vi "CONFIGURE_DIGITIZER_2.vi"(0 "VERTICAL SETTINGS IN":T3, 1 "DIGITIZER 2 CHANNELS":string, 2 "Horizontal Settings IN":T1, 3 "error in":errorcluster, 4 "TRIGGER SETTINGS IN":T2) -> (5 "instrument handle out":refnum<k15>, 6 "error out":errorcluster)   [LabVIEW 2010]
uses:
  <instrlib>/niScope/Controls/niScope trigger slope.ctl
  <instrlib>/niScope/Controls/niScope trigger source.ctl
  <instrlib>/niScope/Controls/niScope trigger source digital.ctl
  <instrlib>/niScope/Configure/Trigger/niScope Configure Trigger Edge.vi
  <instrlib>/niScope/Configure/Trigger/niScope Configure Trigger Digital.vi
  <instrlib>/niScope/Configure/Trigger/niScope Configure Trigger Immediate.vi
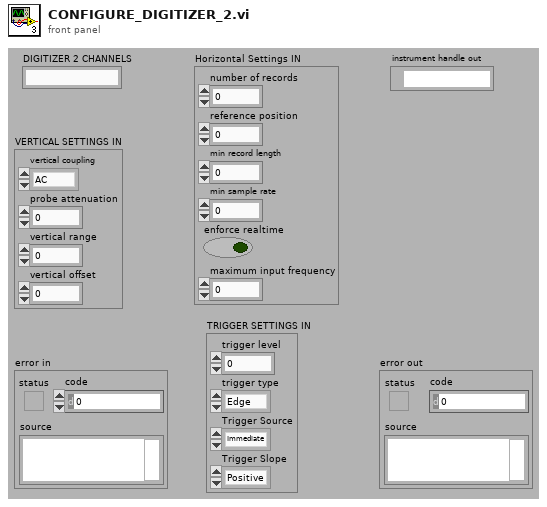
[diagram p1: front panel]
types:
  T1 = cluster{"number of records":i32, "reference position":dbl, "min record length":i32, "min sample rate":dbl, "enforce realtime":bool, "maximum input frequency":dbl}
  T2 = cluster{"trigger level":dbl, "trigger type":enum16{"Edge", "Digital", "Immediate"}, "Trigger Source":enum8{"Immediate", "Channel 0", "Channel 1", "Channel 2", "Channel 3", "Channel 4", "Channel 5", "Channel 6", "Channel 7", "External TRIG", "Software Trigger", "RTSI 0", "RTSI 1", "RTSI 2", "RTSI 3", "RTSI 4", "RTSI 5", "RTSI 6", "PFI 0", "PFI 1", "PFI 2", "PXI Star Trigger"}, "Trigger Slope":enum16{"Positive", "Negative"}}
  T3 = cluster{"vertical coupling":enum16{"AC", "DC", "Ground"}, "probe attenuation":dbl, "vertical range":dbl, "vertical offset":dbl}
  T4 = enum8{"Immediate", "Channel 0", "Channel 1", "Channel 2", "Channel 3", "Channel 4", "Channel 5", "Channel 6", "Channel 7", "External TRIG", "Software Trigger", "RTSI 0", "RTSI 1", "RTSI 2", "RTSI 3", "RTSI 4", "RTSI 5", "RTSI 6", "PFI 0", "PFI 1", "PFI 2", "PXI Star Trigger"}
  T5 = typedef "niScope trigger source.ctl" = string
  T6 = typedef "niScope trigger source digital.ctl" = string
  T7 = typedef "niScope trigger slope.ctl" = i32
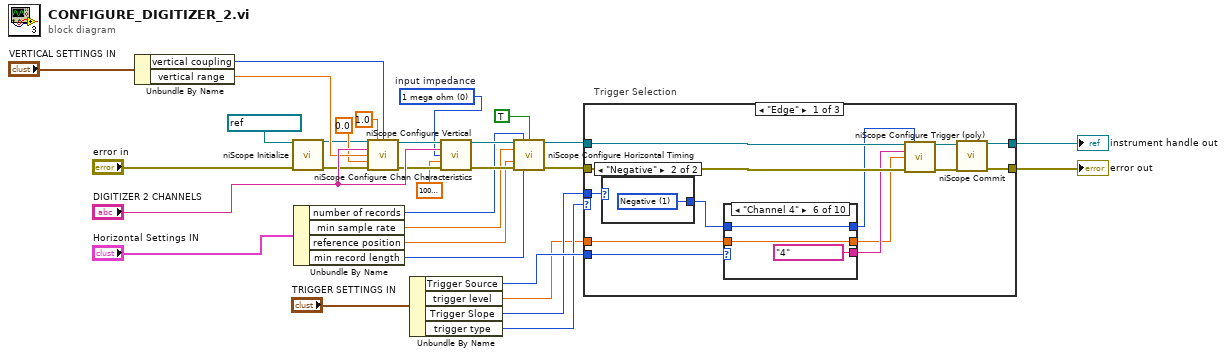
[diagram p0: block diagram]
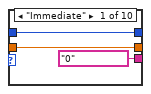
[diagram p2: hidden frame]
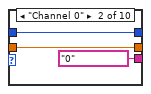
[diagram p3: hidden frame]
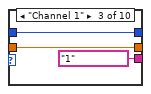
[diagram p4: hidden frame]
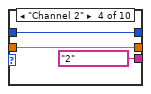
[diagram p5: hidden frame]
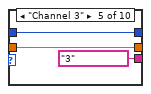
[diagram p6: hidden frame]
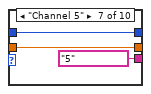
[diagram p7: hidden frame]
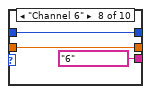
[diagram p8: hidden frame]
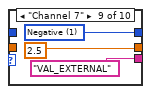
[diagram p9: hidden frame]
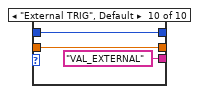
[diagram p10: hidden frame]
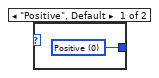
[diagram p11: hidden frame]
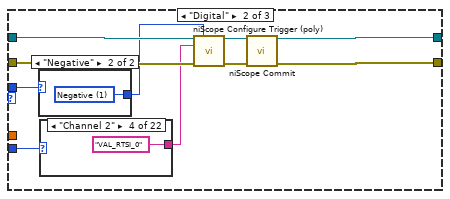
[diagram p12: hidden frame]
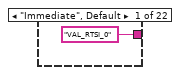
[diagram p13: hidden frame]
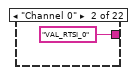
[diagram p14: hidden frame]
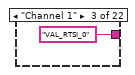
[diagram p15: hidden frame]
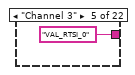
[diagram p16: hidden frame]
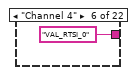
[diagram p17: hidden frame]
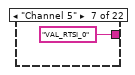
[diagram p18: hidden frame]
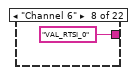
[diagram p19: hidden frame]
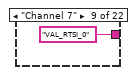
[diagram p20: hidden frame]
diagram:
  w2 = u32 0 items=["1 mega ohm"=0, "50 ohms"=2]  # input impedance
  n1 = Unbundle By Name("VERTICAL SETTINGS IN") -> ("vertical coupling"=w6:enum16{"AC", "DC", "Ground"}, "vertical range"=w26:dbl)
  n2 = call <instrlib>:"niScope Initialize.vi"("resource name"=refnum<k15> "PXI1Slot4", "error in"="error in") -> ("instrument handle"=w3:refnum<k15>, "error out"=w4:errorcluster)  [unwired: 12 in]
  n3 = Unbundle By Name("Horizontal Settings IN") -> ("number of records"=w10:i32, "min sample rate"=w11:dbl, "reference position"=w12:dbl, "min record length"=w13:i32)
  n4 = call <instrlib>:"niScope Configure Vertical.vi"("instrument handle"=w3, "probe attenuation"=1.0, "vertical coupling"=w6, "channels"="DIGITIZER 2 CHANNELS", "vertical range"=w26, "vertical offset"=0.0, "error in"=w4) -> ("instrument handle out"=w27:refnum<k15>, "error out"=w29:errorcluster)  [unwired: 7 in]
  n5 = Unbundle By Name("TRIGGER SETTINGS IN") -> ("Trigger Source"=w24:T4, "trigger level"=w21:dbl, "Trigger Slope"=w23:enum16{"Positive", "Negative"}, "trigger type"=w22:enum16{"Edge", "Digital", "Immediate"})
  n6 = call <instrlib>:"niScope Configure Chan Characteristics.vi"("instrument handle"=w27, "channels"="DIGITIZER 2 CHANNELS", "input impedance"=w2, "maximum input frequency"=10000000.0, "error in"=w29) -> ("instrument handle out"=w28:refnum<k15>, "error out"=w30:errorcluster)  [unwired: 9 in]
  n7 = call <instrlib>:"niScope Configure Horizontal Timing.vi"("instrument handle"=w28, "number of records"=w10, "enforce realtime"=TRUE, "min sample rate"=w11, "reference position"=w12, "error in"=w30, "min record length"=w13) -> ("instrument handle out"=w17:refnum<k15>, "error out"=w20:errorcluster)  [unwired: 7 in]
  n8 = case "Trigger Selection" shown="\"Edge\"" w22 {
    tunnel: w20 -> [w44 w86 w114]
    tunnel: [w36 w77 w111] -> w19
    tunnel: w17 -> [w43 w85 w113]
    tunnel: [w38 w78 w112] -> w18
    tunnel: w24 -> [w41 w82 _]
    tunnel: w21 -> [w35 _ _]
    tunnel: w23 -> [w42 w84 _]
    frame "Edge" {
      n9 = case shown="\"Negative\"" w42 {
        tunnel: [w75 w76] -> w33
        frame "Positive", Default {
          w75 = T7 0 items=["Positive", "Negative"] ("trigger slope")
        }
        frame "Negative" {
          w76 = T7 1 items=["Positive", "Negative"] ("trigger slope")
        }
      }
      n10 = case shown="\"Channel 4\"" w41 {
        tunnel: [T5 "0" ("trigger source") T5 "0" ("trigger source") T5 "1" ("trigger source") T5 "2" ("trigger source") T5 "3" ("trigger source") T5 "4" ("trigger source") T5 "5" ("trigger source") T5 "6" ("trigger source") T5 "VAL_EXTERNAL" ("trigger source") T5 "VAL_EXTERNAL" ("trigger source")] -> w40
        tunnel: w35 -> [w46 w48 w51 w54 w57 w60 w63 w66 _ w72]
        tunnel: [w46 w48 w51 w54 w57 w60 w63 w66 2.5 ("trigger level") w72] -> w34
        tunnel: w33 -> [w45 w49 w52 w55 w58 w61 w64 w67 _ w73]
        tunnel: [w45 w49 w52 w55 w58 w61 w64 w67 w69 w73] -> w32
        frame "Immediate" {
        }
        frame "Channel 0" {
        }
        frame "Channel 1" {
        }
        frame "Channel 2" {
        }
        frame "Channel 3" {
        }
        frame "Channel 4" {
        }
        frame "Channel 5" {
        }
        frame "Channel 6" {
        }
        frame "Channel 7" {
          w69 = T7 1 items=["Positive", "Negative"] ("trigger slope")
        }
        frame "External TRIG", Default {
        }
      }
      n11 = call-poly <instrlib>:"niScope Configure Trigger (poly).vi"("instrument handle"=w43, "trigger slope"=w32, "trigger source"=w40, "trigger level"=w34, "error in"=w44) -> ("instrument handle out"=w39:refnum<k15>, "error out"=w37:errorcluster)  [unwired: 9 in]
      n12 = call <instrlib>:"niScope Commit.vi"("instrument handle"=w39, "error in"=w37) -> ("instrument handle out"=w38:refnum<k15>, "error out"=w36:errorcluster)  [unwired: 12 in]
    }
    frame "Digital" {
      n13 = case shown="\"Negative\"" w84 {
        tunnel: [w109 w110] -> w83
        frame "Positive", Default {
          w109 = T7 0 items=["Positive", "Negative"] ("trigger slope")
        }
        frame "Negative" {
          w110 = T7 1 items=["Positive", "Negative"] ("trigger slope")
        }
      }
      n14 = case shown="\"Channel 2\"" w82 {
        tunnel: [T6 "VAL_RTSI_0" ("trigger source") T6 "VAL_RTSI_0" ("trigger source") T6 "VAL_RTSI_0" ("trigger source") T6 "VAL_RTSI_0" ("trigger source") T6 "VAL_RTSI_0" ("trigger source") T6 "VAL_RTSI_0" ("trigger source") T6 "VAL_RTSI_0" ("trigger source") T6 "VAL_RTSI_0" ("trigger source") T6 "VAL_RTSI_0" ("trigger source") T6 "VAL_RTSI_0" ("trigger source") T6 "VAL_RTSI_0" ("trigger source") T6 "VAL_RTSI_0" ("trigger source") T6 "VAL_RTSI_1" ("trigger source") T6 "VAL_RTSI_2" ("trigger source") T6 "VAL_RTSI_3" ("trigger source") T6 "VAL_RTSI_4" ("trigger source") T6 "VAL_RTSI_5" ("trigger source") T6 "VAL_RTSI_6" ("trigger source") T6 "VAL_PFI_0" ("trigger source") T6 "VAL_PFI_1" ("trigger source") T6 "VAL_PFI_2" ("trigger source") T6 "VAL_PXI_STAR" ("trigger source")] -> w81
        frame "Immediate", Default {
        }
        frame "Channel 0" {
        }
        frame "Channel 1" {
        }
        frame "Channel 2" {
        }
        frame "Channel 3" {
        }
        frame "Channel 4" {
        }
        frame "Channel 5" {
        }
        frame "Channel 6" {
        }
        frame "Channel 7" {
        }
        frame "External TRIG" {
        }
        frame "Software Trigger" {
        }
        frame "RTSI 0" {
        }
        frame "RTSI 1" {
        }
        frame "RTSI 2" {
        }
        frame "RTSI 3" {
        }
        frame "RTSI 4" {
        }
        frame "RTSI 5" {
        }
        frame "RTSI 6" {
        }
        frame "PFI 0" {
        }
        frame "PFI 1" {
        }
        frame "PFI 2" {
        }
        frame "PXI Star Trigger" {
        }
      }
      n15 = call-poly <instrlib>:"niScope Configure Trigger (poly).vi"("instrument handle"=w85, "trigger slope"=w83, "trigger source"=w81, "error in"=w86) -> ("instrument handle out"=w80:refnum<k15>, "error out"=w79:errorcluster)  [unwired: 10 in]
      n16 = call <instrlib>:"niScope Commit.vi"("instrument handle"=w80, "error in"=w79) -> ("instrument handle out"=w78:refnum<k15>, "error out"=w77:errorcluster)  [unwired: 12 in]
    }
    frame "Immediate", Default {
      n17 = call-poly <instrlib>:"niScope Configure Trigger (poly).vi"("instrument handle"=w113, "error in"=w114) -> ("instrument handle out"=w112:refnum<k15>, "error out"=w111:errorcluster)  [unwired: 12 in]
    }
  }
  "error out" <- w19
  "instrument handle out" <- w18
